vi "has_[n].vi"(8 "error in (no error)":errorcluster, 11 "Instrument Command In":string="TRIGger:AND:ENABle {{ON | 1} | {OFF | 0}} ") -> (0 "error out":errorcluster, 2 "Boolean":bool, 3 "Instrument Command Out":string)   [LabVIEW 2018]
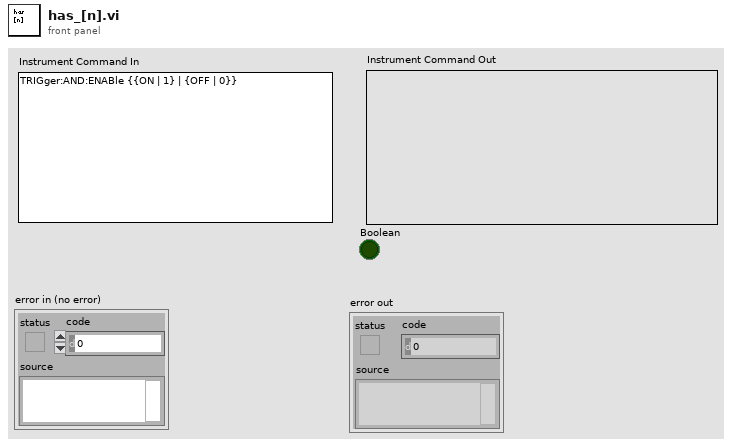
[diagram p1: front panel]
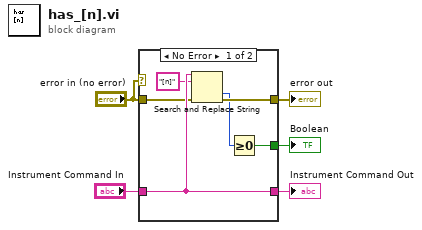
[diagram p0: block diagram]
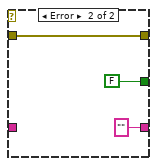
[diagram p2: hidden frame]
diagram:
  n1 = case shown="No Error" "error in (no error)" {
    tunnel: [w11 "" ("result string")] -> w5
    tunnel: "Instrument Command In" -> [w11 _]
    tunnel: "error in (no error)" -> [w9 w13]
    tunnel: [w8 w13] -> w2
    tunnel: [w6 FALSE] -> w1
    frame No Error {
      n2 = Search and Replace String(input string=w11, search string="[n]", error in=w9) -> (offset past replacement=w7:i32, error out=w8:errorcluster)  [unwired: 7 out]
      n3 = Greater Or Equal To 0?(x=w7) -> (x >= 0?=w6:bool)
    }
    frame Error {
    }
  }
  "Instrument Command Out" <- w5
  "error out" <- w2
  "Boolean" <- w1
